vi "PH_SHS_Analysis_Statistician.set i attribute.vi"(0 "i ref in":refnum<vi>, 2 "i attribute":T1={"GUI Refs "={"Status"=refnum, "Result Graph"=refnum, "Mean Data 1"=refnum, "Std Dev Data 1"=refnum, "Mean Data 2"=refnum, "Std Dev Data 2"=refnum, "Mean Data 3"=refnum, "Std Dev Data 3"=refnum, "Dummy Mean"=refnum, "Dummy Std Dev"=refnum, "Export Data"=refnum, "Data 1"=refnum, "Data 2"=refnum, "Data 3"=refnum, "Stat or Trend"=refnum, "Delete"=refnum, "Analyzer"=refnum, "Current Zernike Coefficients"=refnum, "PtV [Lambda]"=refnum, "sample length"=refnum}, "Analyzer"="", "Stat or Trend"=FALSE, "Data 1"=0, "Data 2"=0, "Data 3"=0, "Data"=[], "sample length"=1, "Datasets strored"=0, "Dataarray Size"=0} {"Data"."State" items=["no info", "off/false/out", "on/true/in", "Failure", "Alarm", "Status 1", "Status 2", "Status 3"]; "Data"."Zernicke Coefficients"."2nd Spherical" scale=-2.0..2.0 scale format="%.2f"; "Data"."Zernicke Coefficients"."2nd Coma y" scale=-2.0..2.0 scale format="%.2f"; "Data"."Zernicke Coefficients"."2nd Coma x" scale=-2.0..2.0 scale format="%.2f"; "Data"."Zernicke Coefficients"."2nd Astig 45°" scale=-2.0..2.0 scale format="%.2f"; "Data"."Zernicke Coefficients"."2nd Astig 0°" scale=-2.0..2.0 scale format="%.2f"; "Data"."Zernicke Coefficients"."Trefoil 30°" scale=-2.0..2.0 scale format="%.2f"; "Data"."Zernicke Coefficients"."Trefoil 0°" scale=-2.0..2.0 scale format="%.2f"; "Data"."Zernicke Coefficients"."Spherical" scale=-2.0..2.0 scale format="%.2f"; "Data"."Zernicke Coefficients"."Coma y" scale=-2.0..2.0 scale format="%.2f"; "Data"."Zernicke Coefficients"."Coma x" scale=-2.0..2.0 scale format="%.2f"; "Data"."Zernicke Coefficients"."Astig 45°" scale=-2.0..2.0 scale format="%.2f"; "Data"."Zernicke Coefficients"."Astig 0°" scale=-2.0..2.0 scale format="%.2f"; "Data"."Zernicke Coefficients"."Defocus" scale=-2.0..2.0 scale format="%.2f"; "Data"."Zernicke Coefficients"."Tilt y" scale=-2.0..2.0 scale format="%.2f"; "Data"."Zernicke Coefficients"."Tilt x" scale=-2.0..2.0 scale format="%.2f"}, 5 "error in (no error)":errorcluster) -> (14 "i ref out":refnum<vi>, 19 "error out":errorcluster)   [LabVIEW 2014, in "PH_SHS_Analysis_Statistician.lvlib"]
doc: "Sets the i attribute data of an object.\n\nLicense Agreement for this software:\n\nCopyright (C)\nGesellschaft für Schwerionenforschung, GSI\nPlanckstr. 1\n64291 Darmstadt\nGermany\n\nContact: D.Beck@gsi.de \n\nThis program is free software; you can redistribute it and/or modify it under the terms of the GNU General Public License as published by the Free Software Foundation; either version 2 of the license, or (at your option) any later version.\n\nThis program is distributed in the hope that it will be useful, but WITHOUT ANY WARRANTY; without even the implied warranty of MERCHANTABILITY or FITNESS FOR A PARTICULAR PURPOSE. See the GNU General License for more details (http://www.gnu.org).\n\nGesellschaft für Schwerionenforschung, GSI\nPlanckstr. 1, 64291 Darmstadt, Germany\nFor all questions and ideas contact: M.Richter@gsi.de, H.Brand@gsi.de or D.Beck@gsi.de.\nLast update: 17-JUN-2004"
uses:
  PH_SHS_Analysis_Statistician.lvlib
  PH_SHS_Analysis_Statistician.i attribute.ctl
  PH_SHS_Analysis/PH_SHS_Analysis.Zernike Dataset.ctl
  PH_StatusHandler/PH_StatusHandler.Status.ctl
  PH_SHS_Analysis/PH_SHS_Analysis.Zernike Coefficients.ctl
  PH_SHS_Analysis/PH_SHS_Analysis.lvlib
  PH_StatusHandler/PH_StatusHandler.lvlib
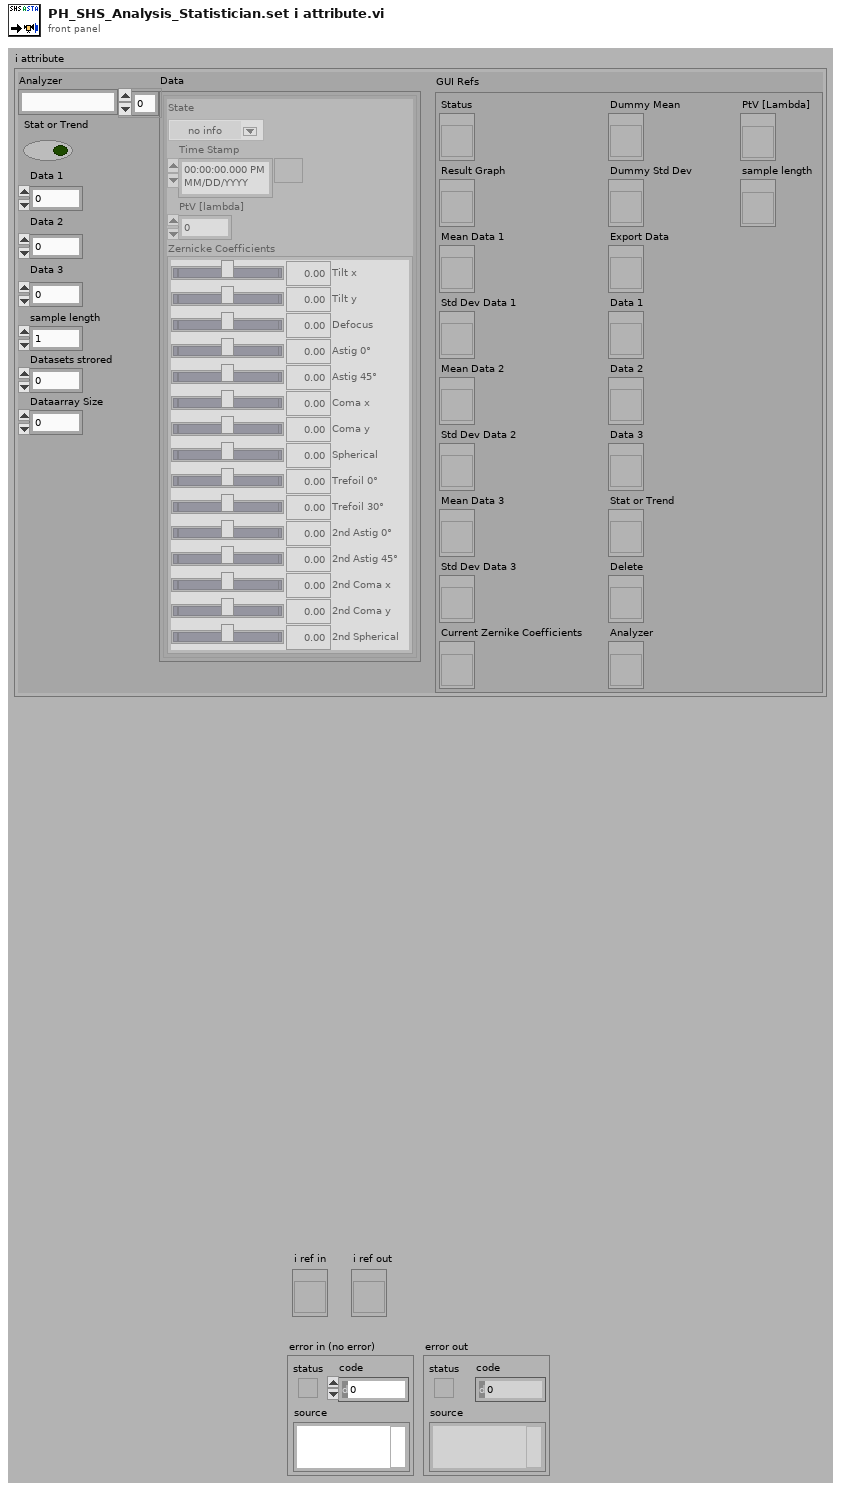
[diagram p1: front panel]
types:
  T1 = typedef "PH_SHS_Analysis_Statistician.lvlib/PH_SHS_Analysis_Statistician.i attribute.ctl" = cluster{"GUI Refs ":cluster{"Status":refnum<vi>, "Result Graph":refnum<vi>, "Mean Data 1":refnum<vi>, "Std Dev Data 1":refnum<vi>, "Mean Data 2":refnum<vi>, "Std Dev Data 2":refnum<vi>, "Mean Data 3":refnum<vi>, "Std Dev Data 3":refnum<vi>, "Dummy Mean":refnum<vi>, "Dummy Std Dev":refnum<vi>, "Export Data":refnum<vi>, "Data 1":refnum<vi>, "Data 2":refnum<vi>, "Data 3":refnum<vi>, "Stat or Trend":refnum<vi>, "Delete":refnum<vi>, "Analyzer":refnum<vi>, "Current Zernike Coefficients":refnum<vi>, "PtV [Lambda]":refnum<vi>, "sample length":refnum<vi>}, "Analyzer":string, "Stat or Trend":bool, "Data 1":i16, "Data 2":i16, "Data 3":i16, "Data":T2[], "sample length":i32, "Datasets strored":i32, "Dataarray Size":i32}
  T2 = typedef "PH_SHS_Analysis.lvlib/PH_SHS_Analysis.Zernike Dataset.ctl" = cluster{"State":T3, "Time Stamp":timestamp, "PtV [lambda]":dbl, "Zernicke Coefficients":T4}
  T3 = typedef "PH_StatusHandler.lvlib/PH_StatusHandler.Status.ctl" = i16
  T4 = typedef "PH_SHS_Analysis.lvlib/PH_SHS_Analysis.Zernike Coefficients.ctl" = cluster{"Tilt x":dbl, "Tilt y":dbl, "Defocus":dbl, "Astig 0°":dbl, "Astig 45°":dbl, "Coma x":dbl, "Coma y":dbl, "Spherical":dbl, "Trefoil 0°":dbl, "Trefoil 30°":dbl, "2nd Astig 0°":dbl, "2nd Astig 45°":dbl, "2nd Coma x":dbl, "2nd Coma y":dbl, "2nd Spherical":dbl}
  T5 = enum16{"SetAttribute", "GetAttribute", "CreateAttribute", "DestroyAttribute", "DestroyAllAtributes"}
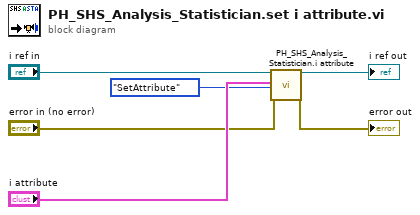
[diagram p0: block diagram]
diagram:
  n1 = call "PH_SHS_Analysis_Statistician.i attribute.vi"("VI Refnum"="i ref in", "CLASS.i attribute"="i attribute", "Action"=T5."SetAttribute", "error in (no error)"="error in (no error)") -> ("VI Refnum out"=→"i ref out":refnum<vi>, "error out"=→"error out":errorcluster)  [unwired: 13 in, 1 out]
